vi "GetDiagramGrowableFunctions.vi"(5 "Diagram":refnum<class "Diagram.lvclass">, 6 "error in":errorcluster, 9 "VI Interpreter in":refnum<class "VI Interpreter.lvclass">) -> (0 "error out":errorcluster, 3 "VI Interpreter out":refnum<class "VI Interpreter.lvclass">, 4 "Diagram out":refnum<class "Diagram.lvclass">)   [LabVIEW 2014, in "Raspberry Pi Compatible Compiler for LabVIEW.lvlib" / "VI Interpreter.lvclass"]
uses:
  VI Interpreter.lvclass
  Diagram/Diagram.lvclass
  Diagram/Diagram.lvclass/Diagram.ctl
  GrowableFunction/GrowableFunction.lvclass
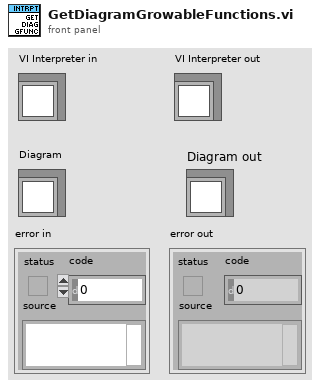
[diagram p1: front panel]
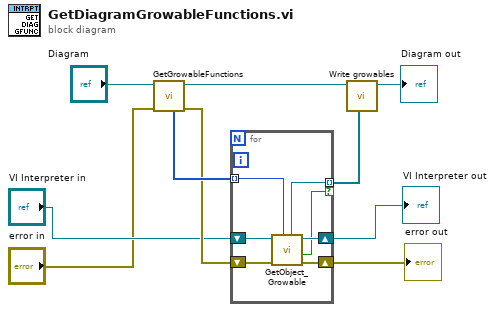
[diagram p0: block diagram]
diagram:
  n1 = call "GetGrowableFunctions.vi"("error in"="error in", "Diagram in"="Diagram") -> ("error out"=w6:errorcluster, "Diagram out"=w1:refnum<class "Diagram.lvclass">, "growable functions"=w7:i32[])  [unwired: 5 in]
  n2 = for {
    shift-right: [w14] -> w10
    shift-left: "VI Interpreter in" -> [w17]
    shift-right: [w16] -> w9
    shift-left: w6 -> [w15]
    tunnel: [w13] -> w3 mode=indexing if=w12
    tunnel: w7 -> [w11] mode=indexing
    n3 = call "GetObject_Growable.vi"("UID"=w11, "error in"=w15, "VI Interpreter in"=w17) -> ("error out"=w16:errorcluster, "found"=w12:bool, "VI Interpreter out"=w14:refnum<class "VI Interpreter.lvclass">, "growable"=w13:refnum<class "GrowableFunction.lvclass">)  [unwired: 3 in]
  }
  "error out" <- w9
  "VI Interpreter out" <- w10
  n4 = call "Write growables.vi"("growables"=w3, "Diagram in"=w1) -> ("Diagram out"=→"Diagram out":refnum<class "Diagram.lvclass">)  [unwired: 7 in]
